vi "SINAD Measurement.vi"() -> ()   [LabVIEW 2023]
doc: "Given an input signal, finds the fundamental frequency and computes Signal, Noise, And Distortion (SINAD). SINAD is defined as the ratio of Signal plus Noise plus Distortion and Noise plus Distortion. You do not need to specify any other input. You can control the amplitude, frequency, and noise level of the input signal. The default signal includes a secondary tone at 11.87 kHz."
uses:
  <vilib>/measure/matone.llb/SINAD Analyzer 1 Chan.vi
  <vilib>/measure/NI_MAPro.lvlib
panel:
  out "SINAD (dB)":dbl
  in  "Fs (Hz)":dbl=51200.0 format="%0.0f"
  in  "signal frequency (Hz)":dbl=1234.89 format="%#.6g"
  in  "amplitude (V)":dbl=1.0 format="%#.6g"
  out "exported time signal":waveform(dbl)(graph)
  in  "Stop":bool
  in  "1mV at 60 Hz":bool
  out "exported signal spectrum (dBV)":T1(graph)
  out "THD Plus Noise (%)":dbl
  in  "block size":i32=1024
  in  "noise \"bitVolt\"":dbl(slide)=-16.018367346938778
  in  "export mode":T2(ring)=enum."input signal"
  out "frequency (Hz)":dbl
  in  "advanced search":T3={"approx freq. (optional)"=-1.0, "search (+/- % of Fsampl.)"=5.0} {"search (+/- % of Fsampl.)" format="%#.6g"; "approx freq. (optional)" format="%#.6g"}
  out "measurement info comments":string
  # "Overview: Demonstrates the use of the SINAD Analyzer VI to find the fundamental tone and associated SINAD (Signal in Noise and Distortion).\nRequirements: LabVIEW Full Development System\nInstructions:\n1. Run the VI and change the noise level slider and note how noise affects  the SINAD measurement.\n2. Use the export mode to select the signal to export.  Try \"residual signal\" to view only the harmonics and noise in the distorted test signal.\n3. Click Stop to stop the VI."
  # "Input Signal"
  # "Analysis Results"
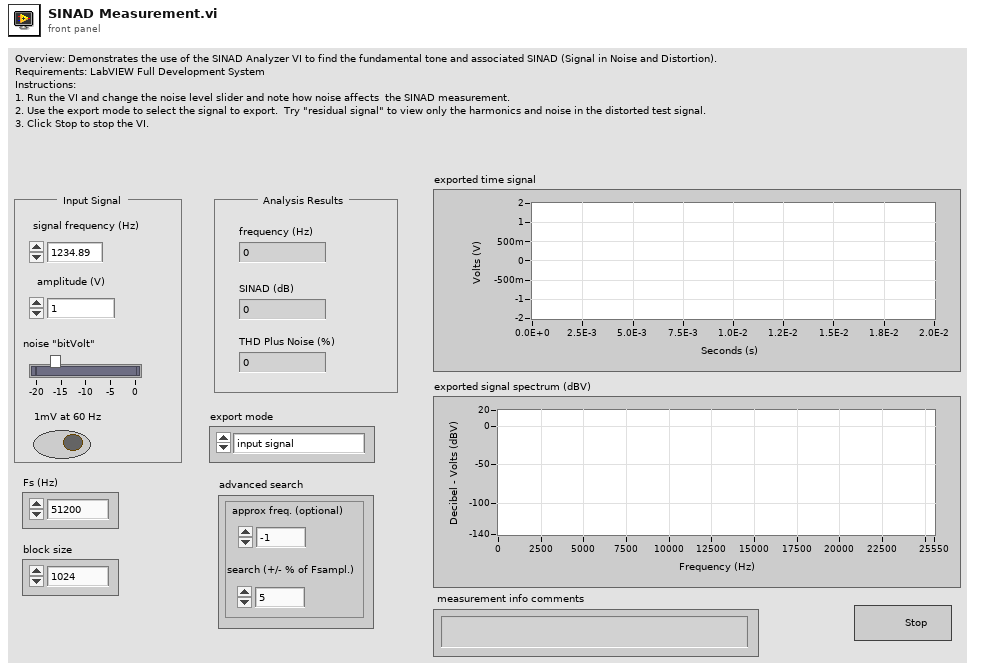
[diagram p1: front panel]
types:
  T1 = cluster{"f0":dbl, "df":dbl, "dB Spectrum (Hann)":dbl[]}
  T2 = enum16{"none", "input signal", "fundamental signal", "residual signal"}
  T3 = cluster{"approx freq. (optional)":dbl, "search (+/- % of Fsampl.)":dbl}
  T4 = cluster{"uncertainty":dbl, "Warning":bool, "comments":string}
  T5 = cluster{"exported time signal":waveform(dbl), "exported spectrum (dB)":cluster{"f0":dbl, "df":dbl, "dB Spectrum (Hann)":dbl[]}}
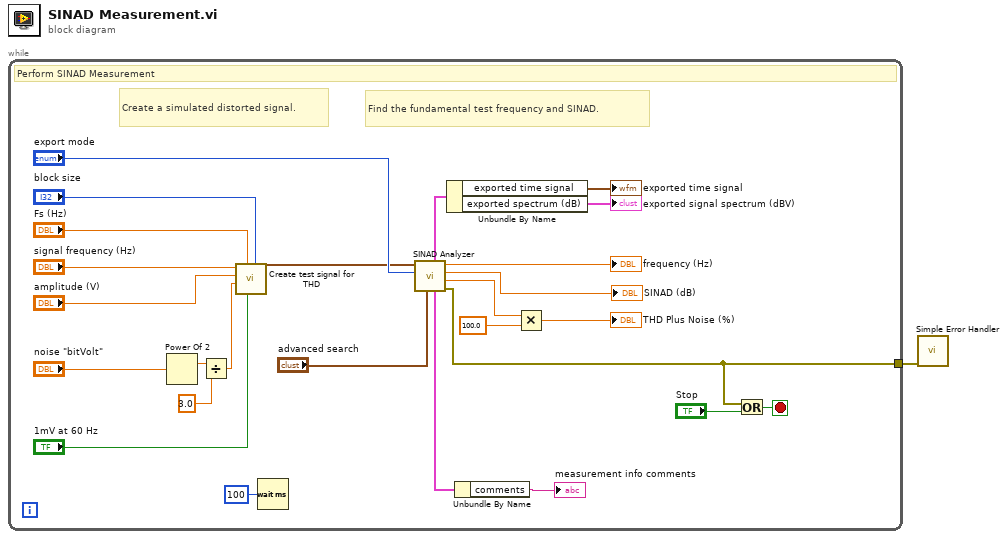
[diagram p0: block diagram]
diagram:
  n1 = while {
    tunnel: [w5] -> w1
    stop <- w10 stop-if-true
    # "Find the fundamental test frequency and SINAD."
    # "Create a simulated distorted signal."
    # "Perform SINAD Measurement"
    n2 = Power Of 2(x="noise \"bitVolt\"") -> (2^x=w25:dbl)
    n3 = Divide(x=w25, y=3.0) -> (x/y=w23:dbl)
    n4 = call "Create test signal for THD.vi"("block size"="block size", "1mV at 60 Hz"="1mV at 60 Hz", "sampling frequency (Hz)"="Fs (Hz)", "noise level (Vrms)"=w23, "fundamental amplitude"="amplitude (V)", "fundamental frequency (Hz)"="signal frequency (Hz)") -> ("Test signal"=w15:waveform(dbl))  [unwired: 5 in]
    n5 = Wait (ms)(milliseconds to wait=u32 100) -> ()  [unwired: 1 out]
    n6 = call-poly <vilib>:"SINAD Analyzer.vi"("advanced search"="advanced search", "export  mode"="export mode", "signal in"=w15) -> ("error out"=w5:errorcluster, "THD Plus Noise"=w8:dbl, "SINAD (dB)"=→"SINAD (dB)":dbl, "detected fundamental\nfrequency"=→"frequency (Hz)":dbl, "measurement info"=w12:T4, "exported signals"=w18:T5)  [unwired: 3 in]
    n7 = Unbundle By Name(w18) -> ("exported time signal"=→"exported time signal":waveform(dbl), "exported spectrum (dB)"=→"exported signal spectrum (dBV)":T1)
    n8 = Unbundle By Name(w12) -> ("comments"=→"measurement info comments":string)
    n9 = Multiply(x=w8, y=100.0) -> (x*y=→"THD Plus Noise (%)":dbl)
    n10 = Or(x=w5, y="Stop") -> (x .or. y?=w10:bool)
  }
  n11 = call <vilib>:"Simple Error Handler.vi"("error in (no error)"=w1) -> ()  [unwired: 4 in, 5 out]
